vi "Document_GetStyleByName.vi"(8 "error in":errorcluster, 10 "StyleName":string, 11 "Document in":refnum<k24>) -> (0 "error out":errorcluster, 2 "Style":refnum<k24>, 3 "Document out":refnum<k24>)   [LabVIEW 2009]
uses:
  C:/Projets/LAVAG/OpenOfficeRGT/AODL/DLLs/AODL.dll
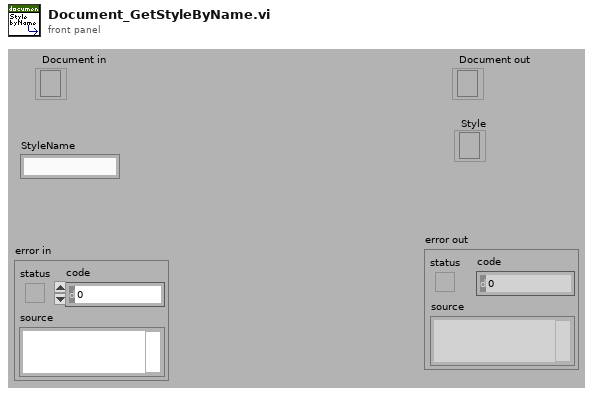
[diagram p1: front panel]
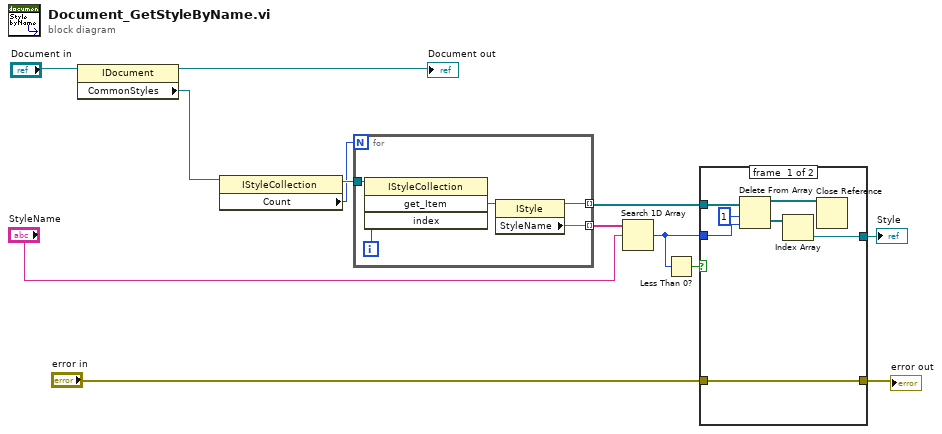
[diagram p0: block diagram]
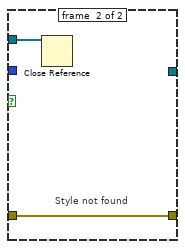
[diagram p2: hidden frame]
diagram:
  n1 = property class="IDocument"(reference="Document in") -> (reference out=→"Document out":refnum<k24>, "CommonStyles"=w11:refnum<k24>)  [unwired: 1 in, 1 out]
  n2 = property class="IStyleCollection"(reference=w11) -> (reference out=w10:refnum<k24>, "Count"=w9:i32)  [unwired: 1 in, 1 out]
  n3 = for {
    N: w9 -> [_]
    tunnel: w10 -> [w18]
    tunnel: [w15] -> w8 mode=indexing
    tunnel: [w14] -> w6 mode=indexing
    i -> [w17]
    n4 = invoke class="IStyleCollection" method="get_Item"(reference=w18, "index"=w17) -> ("get_Item"=w16:refnum<k24>)  [unwired: 2 in, 3 out]
    n5 = property class="IStyle"(reference=w16) -> (reference out=w14:refnum<k24>, "StyleName"=w15:string)  [unwired: 1 in, 1 out]
  }
  n6 = Search 1D Array(1D array=w8, element="StyleName") -> (index of element=w4:i32)  [unwired: 1 in]
  n7 = Less Than 0?(x=w4) -> (x < 0?=w3:bool)
  n8 = case shown="True" w3 {
    tunnel: w6 -> [w25 w27]
    tunnel: [w22 _] -> w5
    tunnel: w4 -> [w20 _]
    tunnel: "error in" -> [w19 w26]
    tunnel: [w19 w26] -> w1
    frame #0 {
      n9 = Delete From Array(array=w25, length=1, index=w20) -> (deleted portion=w23:refnum<k24>[], array with subset deleted=w21:refnum<k24>[])
      n10 = Index Array(array=w23) -> (element=w22:refnum<k24>)  [unwired: 1 in]
      n11 = Close Reference(reference=w21) -> ()  [unwired: 1 in, 1 out]
    }
    frame #1 {
      # "Style not found"
      n12 = Close Reference(reference=w27) -> ()  [unwired: 1 in, 1 out]
    }
  }
  "error out" <- w1
  "Style" <- w5
